vi "Generate Command Sequence.vi"() -> ()   [LabVIEW 2019]
uses:
  Controls/Command Sequene single Control.ctl
  Controls/Command Sequene Control.ctl
panel:
  in  "Auto Control":T1
  out "error out":errorcluster
  out "File path":path
  in  "Path Name":string="paht1"
  out "Command Sequence":string
  in  "Generate Path":bool
  in  "Add Command":bool
  in  "stop":bool
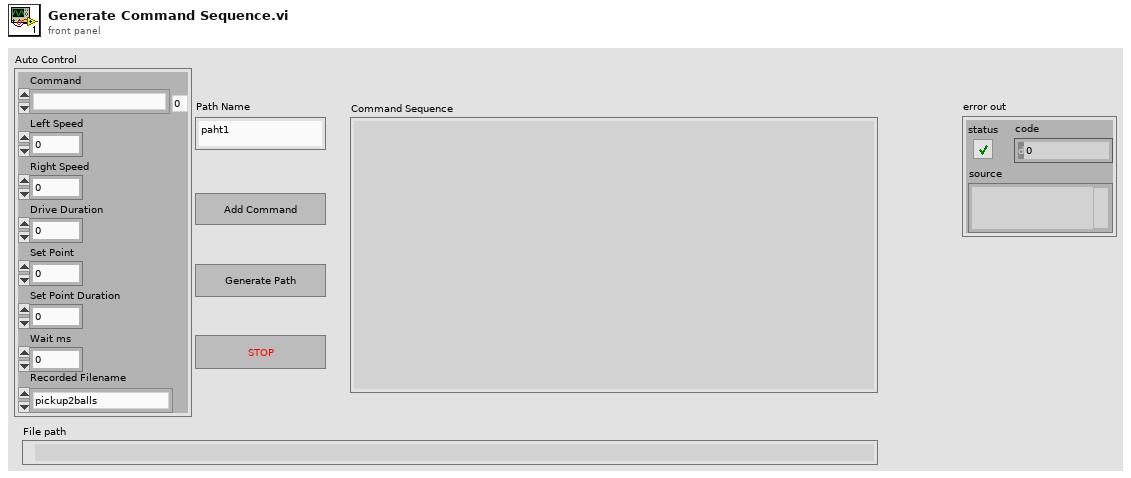
[diagram p1: front panel]
types:
  T1 = typedef "Command Sequene single Control.ctl" = cluster{"Drive Duration":dbl, "Left Speed":dbl, "Right Speed":dbl, "Set Point":dbl, "Set Point Duration":dbl, "Command":enum16{"", "Drive Forwards", "Drive Backwards", "Stop", "Turn Left", "Turn Right", "Drop Intake", "Lift Intake", "Intake", "Shooter", "Transfer", "Wait", "Drive from recorded file"}, "Wait ms":dbl, "Recorded Filename":enum16{"pickup2balls", "drivetoshoot", "pickup5balls", "drivetoshoot5balls"}}
  T2 = typedef "Command Sequene Control.ctl" = enum16{"Idle", "Stop", "Add command", "Create Path File", "Check File Name"}
  T3 = enum16{"open", "replace", "create", "open or create", "replace or create", "replace or create with confirmation"}
  T4 = enum16{"", "Drive Forwards", "Drive Backwards", "Stop", "Turn Left", "Turn Right", "Drop Intake", "Lift Intake", "Intake", "Shooter", "Transfer", "Wait", "Drive from recorded file"}
  T5 = enum16{"pickup2balls", "drivetoshoot", "pickup5balls", "drivetoshoot5balls"}
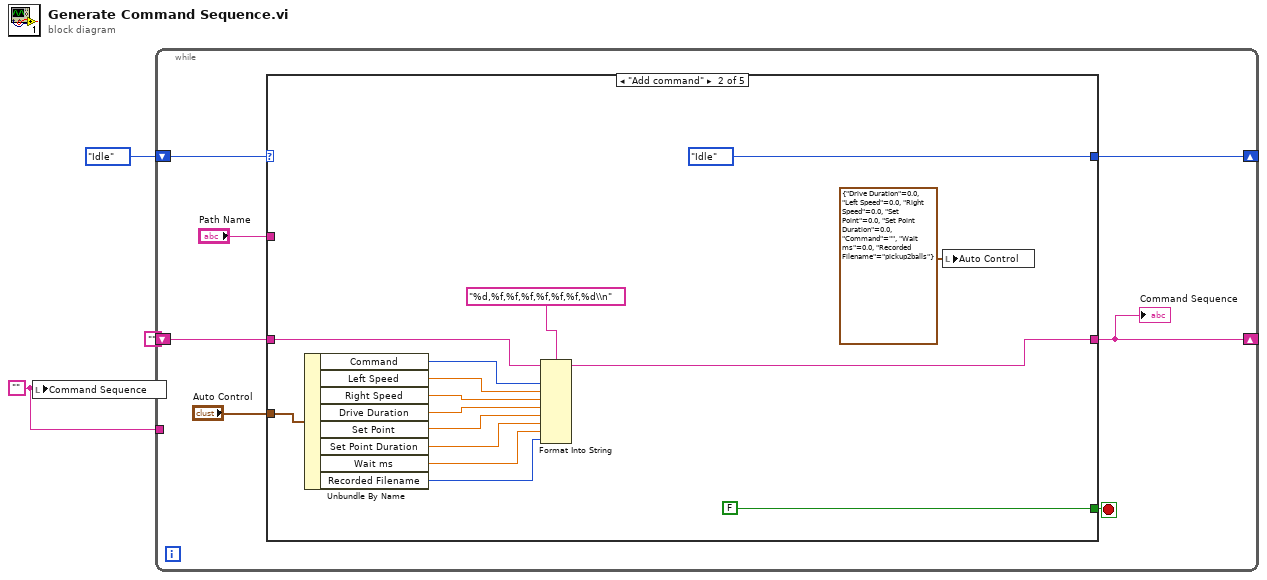
[diagram p0: block diagram]
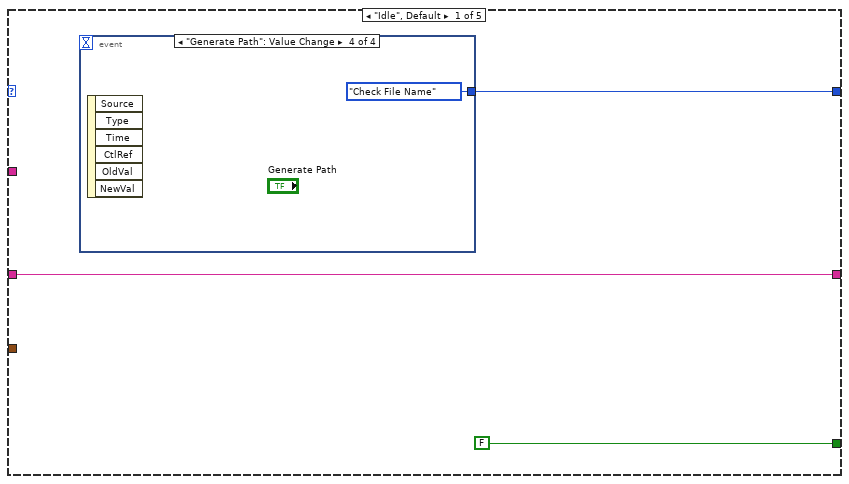
[diagram p2: hidden frame]
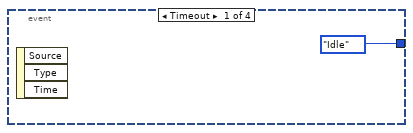
[diagram p3: hidden frame]
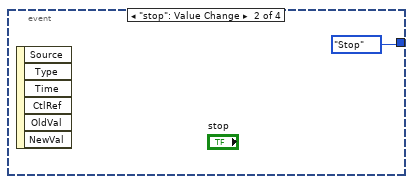
[diagram p4: hidden frame]
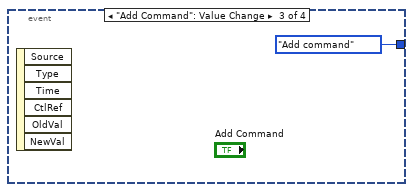
[diagram p5: hidden frame]
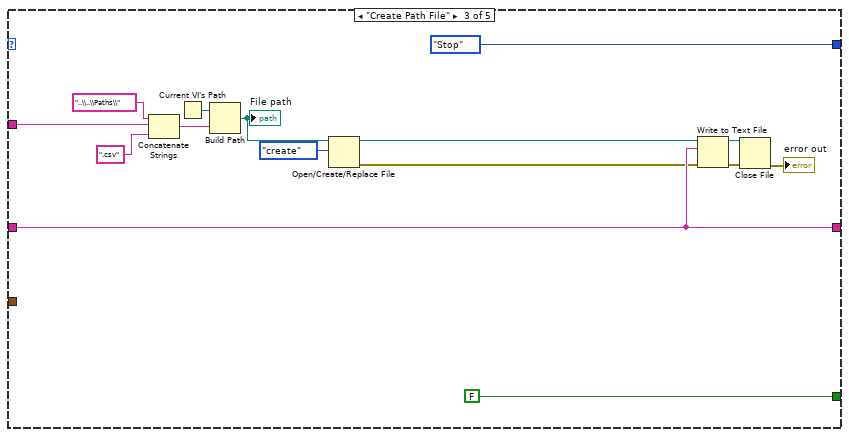
[diagram p6: hidden frame]
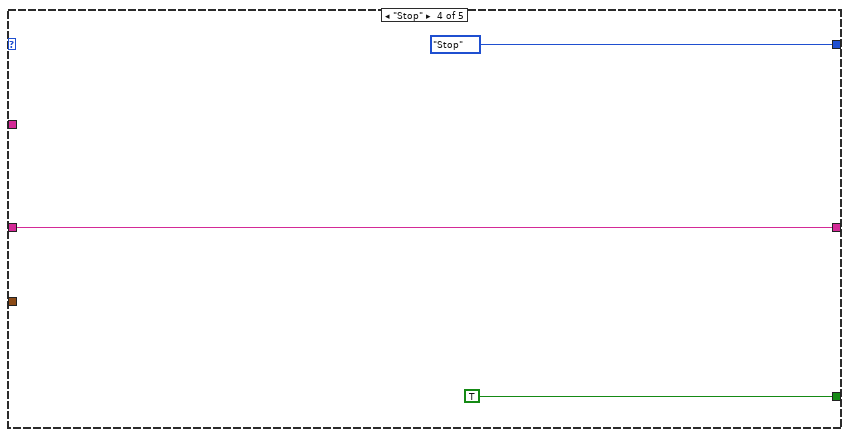
[diagram p7: hidden frame]
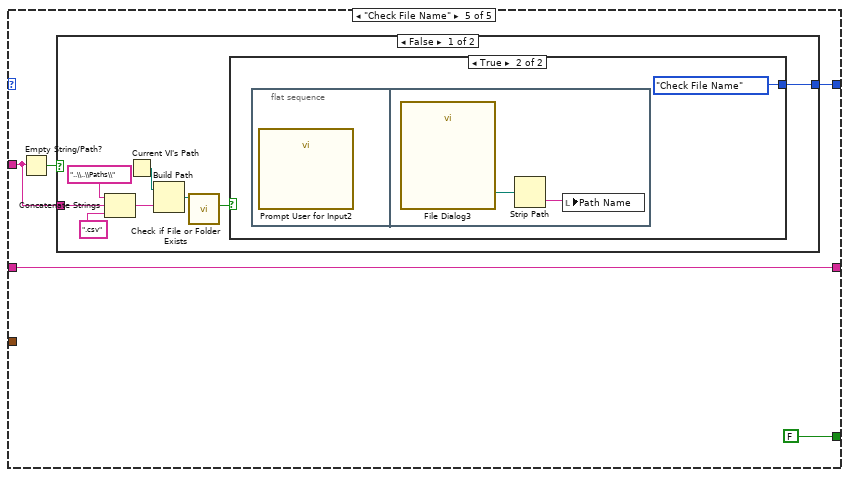
[diagram p8: hidden frame]
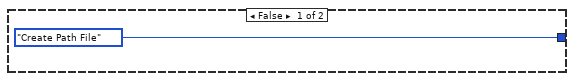
[diagram p9: hidden frame]
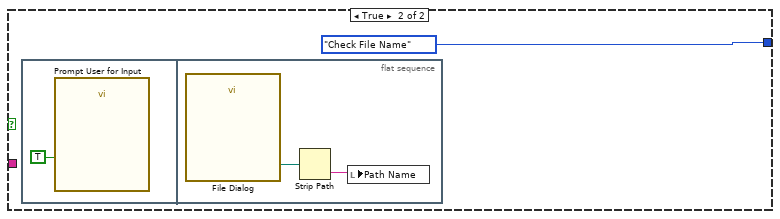
[diagram p10: hidden frame]
diagram:
  w1 = ""
  n1 = local write "Command Sequence"(w1) -> ()
  n2 = while {
    shift-right: [w9] -> _
    shift-left: Command_Sequene_Control."Idle" -> [w10]
    shift-right: [w6] -> _
    shift-left: "" -> [w7]
    tunnel: w1 -> [_]
    stop <- w8 stop-if-true
    n3 = case shown="\"Add command\"" w10 {
      tunnel: [w13 Command_Sequene_Control."Idle" Command_Sequene_Control."Stop" Command_Sequene_Control."Stop" w52] -> w9
      tunnel: [FALSE FALSE FALSE TRUE FALSE] -> w8
      tunnel: "Auto Control" -> [_ w30 _ _ _]
      tunnel: [w11 w21 w45 w48 w54] -> w6
      tunnel: w7 -> [w11 w22 w45 w48 w54]
      tunnel: "Path Name" -> [_ _ w33 _ w51]
      frame "Idle", Default {
        n4 = event shown="[3] \"Generate Path\": Value Change" {
          selector: _ -> [_ _ _ _]
          dyn-events: _ -> [_ _ _ _]
          timeout: _ -> [_ _ _ _]
          tunnel: [Command_Sequene_Control."Idle" Command_Sequene_Control."Stop" Command_Sequene_Control."Add command" Command_Sequene_Control."Check File Name"] -> w13
          event Timeout {
            n5 = event-data() -> ()  [unwired: 1 in, 3 out]
          }
          event "stop": Value Change {
            n6 = event-data() -> ()  [unwired: 1 in, 6 out]
          }
          event "Add Command": Value Change {
            n7 = event-data() -> ()  [unwired: 1 in, 6 out]
          }
          event "Generate Path": Value Change {
            n8 = event-data() -> ()  [unwired: 1 in, 6 out]
          }
        }
      }
      frame "Add command" {
        n9 = Unbundle By Name(w30) -> ("Command"=w28:T4, "Left Speed"=w27:dbl, "Right Speed"=w26:dbl, "Drive Duration"=w25:dbl, "Set Point"=w24:dbl, "Set Point Duration"=w23:dbl, "Wait ms"=w20:dbl, "Recorded Filename"=w18:T5)
        n10 = Format Into String(format string="%d,%f,%f,%f,%f,%f,%f,%d\\n", initial string=w22, w28, w27, w26, w25, w24, w23, w20, w18) -> (resulting string=w21:string)  [unwired: 1 in, 1 out]
        n11 = local write "Auto Control"(T1 {"Drive Duration"=0.0, "Left Speed"=0.0, "Right Speed"=0.0, "Set Point"=0.0, "Set Point Duration"=0.0, "Command"=enum."", "Wait ms"=0.0, "Recorded Filename"=enum."pickup2balls"} ("Auto Control")) -> ()
      }
      frame "Create Path File" {
        n12 = Concatenate Strings("..\\..\\Paths\\" ("string"), w33, ".csv" ("string")) -> (w42:string)
        n13 = Current VI's Path() -> (path=w41:path)
        n14 = Build Path(base path=w41, name or relative path=w42) -> (appended path=w40:path)
        "File path" <- w40
        n15 = Open/Create/Replace File(file path (use dialog)=w40, operation (0:open)=T3."create") -> (refnum out=w36:refnum<file>, error out=w35:errorcluster)  [unwired: 4 in, 1 out]
        n16 = Write to Text File(file (use dialog)=w36, text=w45, error in=w35) -> (refnum out=w44:refnum<file>, error out=w43:errorcluster)  [unwired: 1 in, 1 out]
        n17 = Close File(refnum=w44, error in=w43) -> (error out=→"error out":errorcluster)  [unwired: 1 out]
      }
      frame "Stop" {
      }
      frame "Check File Name" {
        n18 = Empty String/Path?(string/path=w51) -> (empty?=w53:bool)
        n19 = case shown="False" w53 {
          tunnel: [w56 Command_Sequene_Control."Check File Name"] -> w52
          tunnel: w51 -> [w59 _]
          frame False {
            n20 = Concatenate Strings("..\\..\\Paths\\" ("string"), w59, ".csv" ("string")) -> (w63:string)
            n21 = Current VI's Path() -> (path=w62:path)
            n22 = Build Path(base path=w62, name or relative path=w63) -> (appended path=w58:path)
            n23 = call <vilib>:"Check if File or Folder Exists.vi"("path"=w58) -> ("file or folder exists?"=w57:bool)  [unwired: 8 in, 2 out]
            n24 = case shown="True" w57 {
              tunnel: [Command_Sequene_Control."Create Path File" Command_Sequene_Control."Check File Name"] -> w56
              frame False {
              }
              frame True {
                n25 = flat-sequence {
                  frame #0 {
                    n26 = call "Prompt User for Input2"() -> ()  [unwired: 20 in]
                  }
                  frame #1 {
                    n27 = call "File Dialog3"() -> ("selected path"=w67:path)  [unwired: 12 in, 3 out]
                    n28 = Strip Path(path=w67) -> (name=w66:string)  [unwired: 1 out]
                    n29 = local write "Path Name"(w66) -> ()
                  }
                }
              }
            }
          }
          frame True {
            n30 = flat-sequence {
              frame #0 {
                n31 = call "Prompt User for Input"("Enable"=TRUE) -> ()  [unwired: 19 in]
              }
              frame #1 {
                n32 = call "File Dialog"() -> ("selected path"=w71:path)  [unwired: 12 in, 3 out]
                n33 = Strip Path(path=w71) -> (name=w70:string)  [unwired: 1 out]
                n34 = local write "Path Name"(w70) -> ()
              }
            }
          }
        }
      }
    }
    "Command Sequence" <- w6
  }
